vi "findDevice.vi"(8 "error in (no error)":errorcluster, 9 "S/N:":string, 10 "Device Type:":T1=enum."k4b2", 11 "reference in":refnum<class "Devices Controller.lvclass">) -> (0 "error out":errorcluster, 1 "found!":bool, 2 "index of element":i32, 3 "reference out":refnum<class "Devices Controller.lvclass">)   [LabVIEW 2016, in "Devices Controller.lvclass"]
uses:
  Devices Controller.lvclass
  deviceType.ctl
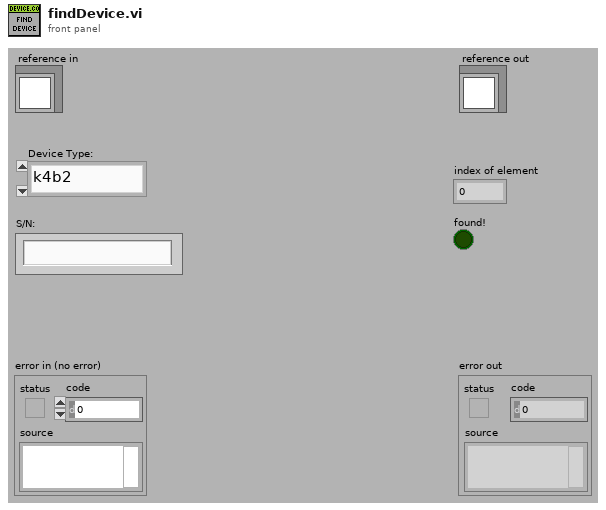
[diagram p1: front panel]
types:
  T1 = typedef "Devices Controller.lvclass/deviceType.ctl" = enum16{"k5", "k4b2", "fitmate", "cpet", "rmr", "bodyBoxPft", "bp", "pp"}
  T2 = typedef "Devices Controller.lvclass/ObjectAttributesRef.ctl" = refnum<data-value>
  T3 = typedef "Devices Controller.lvclass/ObjectAttributes.ctl" = cluster{"MyAttribute":dbl, "file_controller_ref":refnum<class "File Controller.lvclass">, "data":string[][][], "devices_refs":cluster{"k4b2_refs":refnum<class "k4b2.lvclass">[], "rmr_refs":refnum<class "rmr.lvclass">[], "bod_pod_refs":refnum<class "bodpod.lvclass">[], "cpet_refs":refnum<class "cpet.lvclass">[], "fitmate_refs":refnum<class "fitmate.lvclass">[], "pea_pod_refs":refnum<class "peapod.lvclass">[], "k5_refs":refnum<class "k5.lvclass">[], "bb-pft_refs":refnum<class "bb-pft.lvclass">[]}}
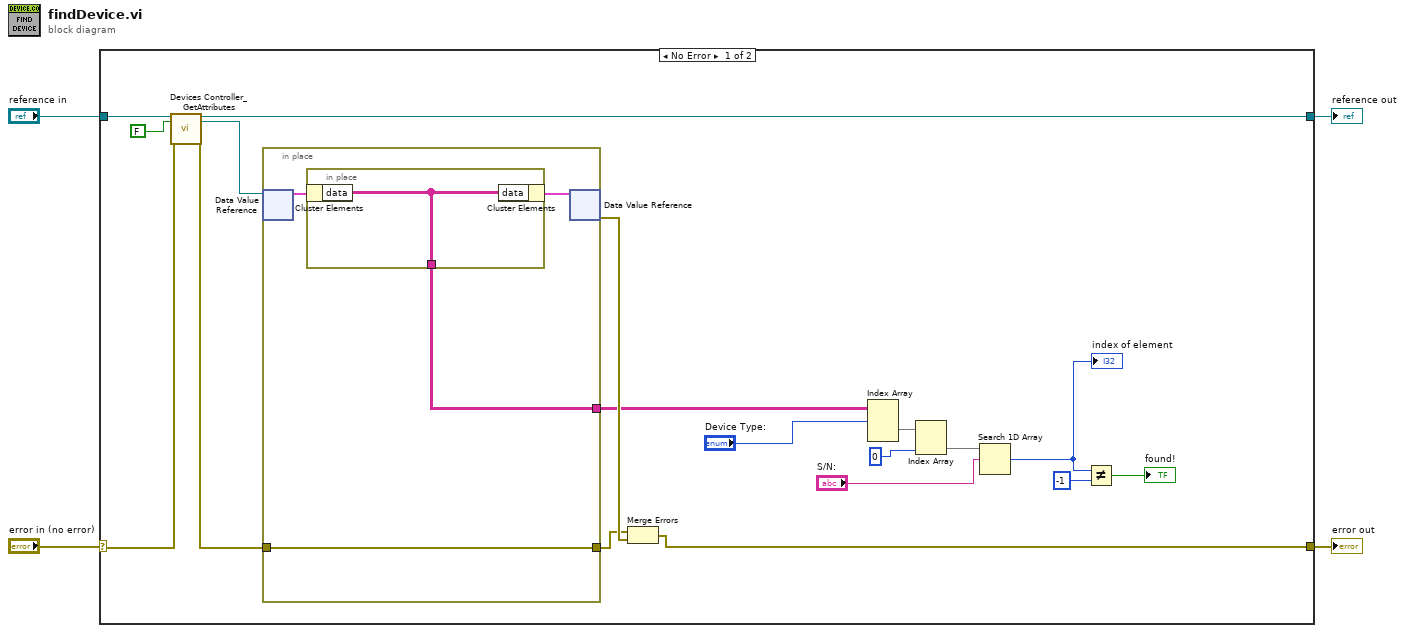
[diagram p0: block diagram]
diagram:
  n1 = case shown="No Error" "error in (no error)" {
    selector: "error in (no error)" -> [w17 w29]
    tunnel: [w22 w29] -> w3
    tunnel: [w15 w28] -> w1
    tunnel: "reference in" -> [w19 w28]
    frame No Error {
      n2 = call "Devices Controller_GetAttributes.vi"("reference in"=w19, "return data? (T)"=FALSE, "error in (no error)"=w17) -> ("reference out"=w15:refnum<class "Devices Controller.lvclass">, "attributes ref"=w14:T2, "error out"=w16:errorcluster)  [unwired: 13 in, 1 out]
      n3 = in-place {
        in-place-border: w16 -> [w24]
        in-place-border: [w24] -> w20
        in-place-border: [w23] -> w9
        n4 = in-place-dvr #1(w14) -> (w25:T3)  [unwired: 1 out]
        n5 = in-place {
          in-place-border: [w27] -> w23
          n6 = in-place-cluster #2(w25) -> ("data"=w27:string[][][])
          n7 = in-place-cluster #2("data"=w27) -> (w26:T3)
        }
        n8 = in-place-dvr #1(w26) -> (w21:errorcluster)  [unwired: 1 out]
      }
      n9 = Merge Errors(w20, w21) -> (w22:errorcluster)
      n10 = Index Array(array=w9, index (dim 0)="Device Type:") -> (element=w13:string[][])  [unwired: 2 in]
      n11 = Index Array(array=w13, index (col)=0 ("disabled index (col)")) -> (element=w11:string[])  [unwired: 1 in]
      n12 = Search 1D Array(1D array=w11, element="S/N:") -> (index of element=w8:i32)  [unwired: 1 in]
      "index of element" <- w8
      n13 = Not Equal?(x=w8, y=-1) -> (x != y?=→"found!":bool)
    }
    frame Error {
    }
  }
  "error out" <- w3
  "reference out" <- w1
